vi "Config - CloseConnection.vi"(8 "Fehler (Eingang, kein Fehler)":errorcluster) -> (0 "Fehler (Ausgang)":errorcluster)   [LabVIEW 2016]
uses:
  eGateUtility.dll
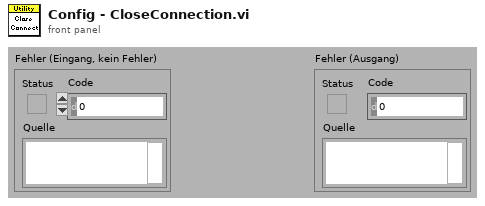
[diagram p1: front panel]
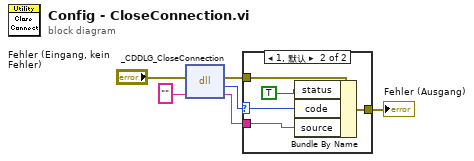
[diagram p0: block diagram]
diagram:
  n1 = dll-call lib="eGateUtility.dll" fn="_CDDLG_CloseConnection"(error in="Fehler (Eingang, kein Fehler)", "ErrorString"="") -> (error out=w4:errorcluster, "Rückgabetyp"=w1:i32, "ErrorString"=w2:string)  [unwired: 2 in, 1 out]
  n2 = case shown="1, 默认" w1 {
    selector: w1 -> [_ w9]
    tunnel: w4 -> [w7 w12]
    tunnel: [w7 w11] -> w3
    tunnel: w2 -> [_ w10]
    frame 0 {
    }
    frame 1, Default {
      n3 = Bundle By Name(cluster=w12, "status"=TRUE, "code"=w9, "source"=w10) -> (w11:errorcluster)
    }
  }
  "Fehler (Ausgang)" <- w3
